vi "Table Initialize_1D.vi"(4 "행의 개수":u32, 5 "Table Ref":refnum<vi>, 6 "Value":string[](array[string]), 7 "비활성화?":bool, 8 "에러 입력":errorcluster caption="에러 입력(에러 없음)", 9 "열해더 문자열":string[](array[string]), 10 "열의 개수":u32, 11 "최상단보기?":bool) -> (0 "에러 출력":errorcluster, 1 "Bottom":i32, 3 "Table Ref out":refnum<vi>)   [LabVIEW 2020]
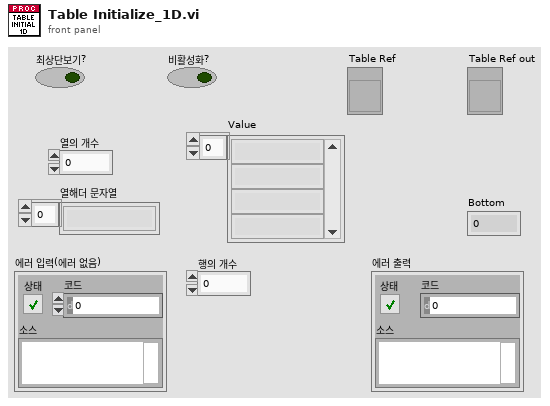
[diagram p1: front panel]
types:
  T1 = enum8{"Enabled", "Disabled", "Disabled and Grayed Out"}
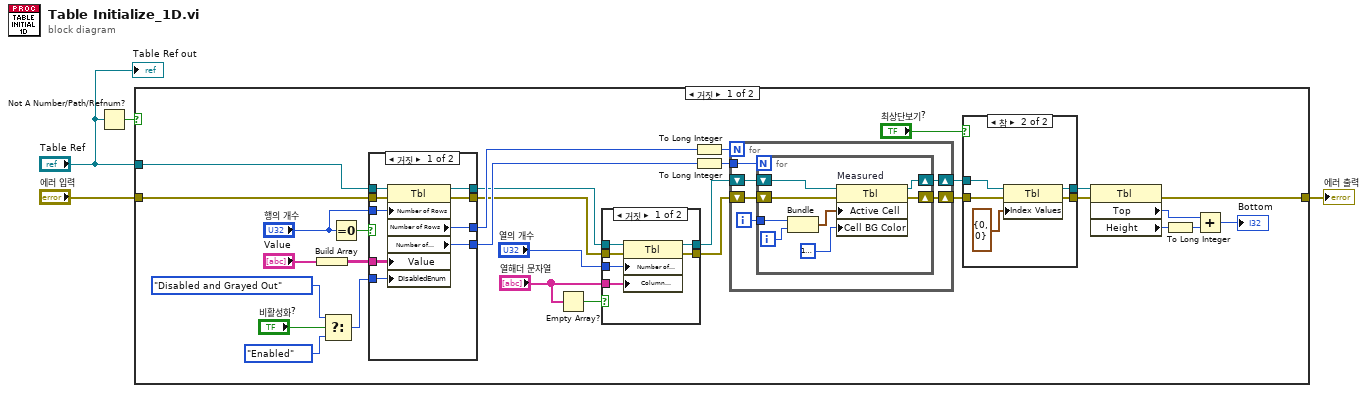
[diagram p0: block diagram]
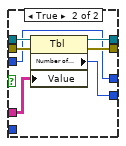
[diagram p4: hidden frame]
diagram:
  n1 = Not A Number/Path/Refnum?(number/path/refnum="Table Ref") -> (NaN/Path/Refnum?=w1:bool)
  n2 = case shown="거짓" w1 {
    tunnel: "에러 입력" -> [w33 w79]
    tunnel: "Table Ref" -> [w27 _]
    tunnel: [w21 w79] -> w3
    frame False {
      n3 = Build Array("Value") -> (w5:string[][])
      n4 = Select(t=T1."Disabled and Grayed Out" ("비활성화"), s="비활성화?", f=T1."Enabled" ("비활성화")) -> (s? t:f=w13:T1)
      n5 = Equal To 0?(x="행의 개수") -> (x = 0?=w25:bool)
      n6 = case shown="거짓" w25 {
        tunnel: w33 -> [w57 w64]
        tunnel: w5 -> [w56 w63]
        tunnel: [w55 w62] -> w10
        tunnel: [w54 w61] -> w31
        tunnel: [w53 w60] -> w9
        tunnel: [w52 w58] -> w28
        tunnel: w27 -> [w51 w59]
        tunnel: "행의 개수" -> [w50 w58]
        tunnel: w13 -> [w49 _]
        frame False {
          n7 = property class="Tbl"(reference=w51, error in=w57, "Number of Rows"=w50, "Value"=w56, "DisabledEnum"=w49) -> (reference out=w53:refnum<vi>, error out=w55:errorcluster, "Number of Rows"=w52:u32, "Number of Columns"=w54:u32)
        }
        frame True {
          n8 = property class="Tbl"(reference=w59, error in=w64, "Value"=w63) -> (reference out=w60:refnum<vi>, error out=w62:errorcluster, "Number of Columns"=w61:u32)
        }
      }
      n9 = Empty Array?(array="열해더 문자열") -> (empty?=w6:bool)
      n10 = case shown="거짓" w6 {
        tunnel: w10 -> [w39 w40]
        tunnel: [w38 w40] -> _
        tunnel: [w37 w41] -> _
        tunnel: w9 -> [w36 w41]
        tunnel: "열의 개수" -> [w35 _]
        tunnel: "열해더 문자열" -> [w34 _]
        frame False {
          n11 = property class="Tbl"(reference=w36, error in=w39, "Number of Columns"=w35, "Column Headers[]"=w34) -> (reference out=w37:refnum<vi>, error out=w38:errorcluster)
        }
        frame True {
        }
      }
      n12 = To Long Integer(number=w28) -> (32bit integer=w30:i32)
      n13 = To Long Integer(number=w31) -> (32bit integer=w29:i32)
      n14 = for {
        N: w30 -> [_]
        shift-right: [w68] -> w24
        shift-left: w10 -> [w69]
        tunnel: w29 -> [w66]
        shift-right: [w65] -> w22
        shift-left: w9 -> [w70]
        i -> [w67]
        n15 = for {
          N: w66 -> [_]
          shift-right: [w76] -> w68
          shift-left: w69 -> [w77]
          tunnel: w67 -> [w75]
          shift-right: [w71] -> w65
          shift-left: w70 -> [w78]
          i -> [w74]
          n16 = Bundle(w75, w74) -> (w73:cluster{i32, i32})  [unwired: 1 in]
          n17 = property on="Measured" class="Tbl"(reference=w78, error in=w77, "Active Cell"=w73, "Cell BG Color"=u32 16777226) -> (reference out=w71:refnum<vi>, error out=w76:errorcluster)
        }
      }
      n18 = case shown="참" "최상단보기?" {
        tunnel: w24 -> [w43 w48]
        tunnel: [w43 w47] -> w12
        tunnel: w22 -> [w42 w46]
        tunnel: [w42 w44] -> w11
        frame False {
        }
        frame True {
          n19 = property class="Tbl"(reference=w46, error in=w48, "Index Values"=cluster{"Row":u32, "Column":u32} {"Row"=0, "Column"=0} ("인덱스 값")) -> (reference out=w44:refnum<vi>, error out=w47:errorcluster)
        }
      }
      n20 = property class="Tbl"(reference=w11, error in=w12) -> (error out=w21:errorcluster, "Top"=w19:i32, "Height"=w18:u32)  [unwired: 1 out]
      n21 = To Long Integer(number=w18) -> (32bit integer=w20:i32)
      n22 = Add(x=w19, y=w20) -> (x+y=→"Bottom":i32)
    }
    frame True {
    }
  }
  "에러 출력" <- w3
  "Table Ref out" <- "Table Ref"
